vi "Test Piccolo Hist Conversion.vi"() -> ()   [LabVIEW 2021, in "Piccolo.lvlib"]
uses:
  <vilib>/Utility/error.llb/Error Cluster From Error Code.vi
  <vilib>/ErrorRing/Error Ring.xnode
  Piccolo.lvlib
panel:
  in  "Gate":u8
  out "Intensity Graph":u16[][](graph)
  in  "Pixel Y":u8 max=31
  in  "Pixel X":u8 max=31
  out "Waveform Graph":u16[](graph)
  out "Data":u16[][][](array[numeric])
  out "cancelled":bool
  out "Error Out":errorcluster
  in  "Error In":errorcluster
  in  "File Path":path
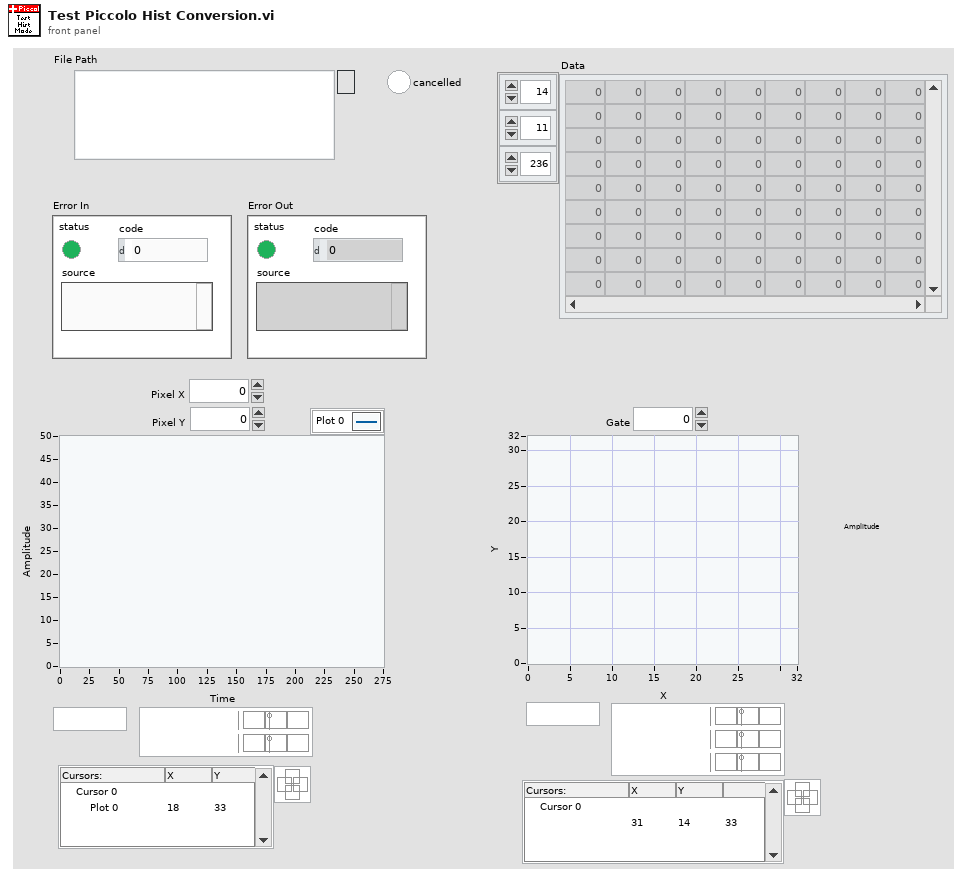
[diagram p1: front panel]
types:
  T1 = enum16{"big-endian, network order", "native, host order", "little-endian"}
  T2 = enum16{"open", "replace", "create", "open or create", "replace or create", "replace or create with confirmation"}
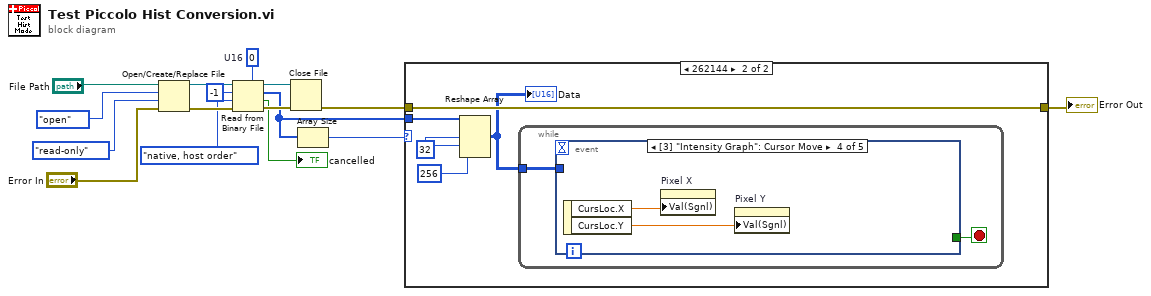
[diagram p0: block diagram]
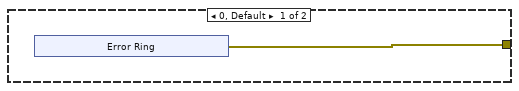
[diagram p2: hidden frame]
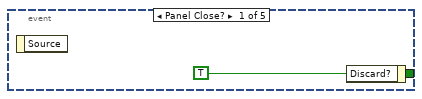
[diagram p3: hidden frame]
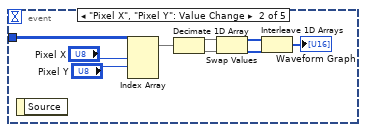
[diagram p4: hidden frame]
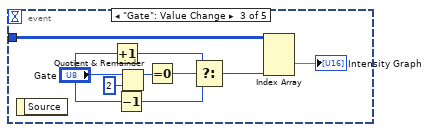
[diagram p5: hidden frame]
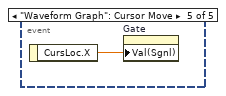
[diagram p6: hidden frame]
diagram:
  w10 = u16 0  # U16
  n1 = Open/Create/Replace File(file path (use dialog)="File Path", error in="Error In", operation (0:open)=T2."open", access (0:read/write)=enum16{"read/write", "read-only", "write-only"}."read-only") -> (refnum out=w12:refnum<file>, error out=w11:errorcluster)  [unwired: 2 in, 1 out]
  n2 = Read from Binary File(5:w10, 8:w11, 9:T1."native, host order" ("byte order (0:big-endian, network order)"), 10:-1 ("count (1)"), 11:w12) -> (0:w8:errorcluster, 1:→"cancelled":bool, 2:w4:u16[], 3:w9:refnum<file>)  [unwired: 1 in]
  n3 = Close File(refnum=w9, error in=w8) -> (error out=w3:errorcluster)  [unwired: 1 out]
  n4 = Array Size(array=w4) -> (size(s)=w5:i32)
  n5 = case shown="262144" w5 {
    tunnel: w4 -> [_ w26]
    tunnel: w3 -> [_ w25]
    tunnel: [w17 w25] -> w2
    frame 0, Default {
      n6 = xnode "Error Ring"() -> ("error out"=w17:errorcluster)
    }
    frame 262144 {
      w23 = 32 ("dimension size")
      n7 = Reshape Array(w26, w23, w23, 256 ("dimension size")) -> (w24:u16[][][])
      "Data" <- w24
      n8 = while {
        tunnel: w24 -> [w27]
        stop <- w28 stop-if-true
        n9 = event shown="[3] \"Intensity Graph\": Cursor Move" {
          selector: _ -> [_ _ _ _ _]
          dyn-events: _ -> [_ _ _ _ _]
          timeout: _ -> [_ _ _ _ _]
          tunnel: [w29 _ _ _ _] -> w28
          tunnel: w27 -> [_ w38 w47 _ _]
          event Panel Close? {
            w29 = TRUE ("Discard?")
            n10 = event-data() -> ()  [unwired: 1 in, 1 out]
            n11 = event-data("Discard?"=w29) -> ()  [unwired: 1 in, 1 out]
          }
          event "Pixel X", "Pixel Y": Value Change {
            n12 = event-data() -> ()  [unwired: 1 in, 1 out]
            n13 = Index Array(array=w38, index (dim 0)="Pixel X", index (dim 1)="Pixel Y") -> (element=w37:u16[])  [unwired: 1 in]
            n14 = Decimate 1D Array(w37) -> (w33:u16[], w32:u16[])
            n15 = Swap Values(12:w33, 14:w32) -> (1:w31:u16[], 3:w30:u16[])  [unwired: 1 in]
            n16 = Interleave 1D Arrays(w31, w30) -> (→"Waveform Graph":u16[])
          }
          event "Gate": Value Change {
            n17 = event-data() -> ()  [unwired: 1 in, 1 out]
            n18 = Increment(x="Gate") -> (x+1=w40:u8)
            n19 = Decrement(x="Gate") -> (x-1=w39:u8)
            n20 = Quotient & Remainder(x="Gate", y=u8 2) -> (x-y*floor(x/y)=w45:u8)  [unwired: 1 out]
            n21 = Equal To 0?(x=w45) -> (x = 0?=w44:bool)
            n22 = Select(t=w40, s=w44, f=w39) -> (s? t:f=w42:u8)
            n23 = Index Array(array=w47, index (dim 2)=w42) -> (element=→"Intensity Graph":u16[][])  [unwired: 2 in]
          }
          event "Intensity Graph": Cursor Move {
            n24 = event-data() -> ("CursLoc.X"=w49:dbl, "CursLoc.Y"=w48:dbl)  [unwired: 1 in]
            n25 = property on="Pixel X" class="DigNum (strict)"("Val(Sgnl)"=w49) -> ()  [unwired: 2 in, 2 out]
            n26 = property on="Pixel Y" class="DigNum (strict)"("Val(Sgnl)"=w48) -> ()  [unwired: 2 in, 2 out]
          }
          event "Waveform Graph": Cursor Move {
            n27 = event-data() -> ("CursLoc.X"=w50:dbl)  [unwired: 1 in]
            n28 = property on="Gate" class="DigNum (strict)"("Val(Sgnl)"=w50) -> ()  [unwired: 2 in, 2 out]
          }
        }
      }
    }
  }
  "Error Out" <- w2
